vi "与其他模块交互 (子VI).vi"() -> ()   [LabVIEW 2016, in "质控单元.lvlib"]
uses:
  <vilib>/Plasmionique/MB Master/MB_Master_TCP/MB_Master_TCP.lvclass
  D:/Program Files (x86)/National Instruments/LabVIEW 2016/vi.lib/Plasmionique/MB Master/MB_Master/MB_Master.lvclass
  <vilib>/Plasmionique/MB Master/MB_Master/MB_Master.lvclass
  <vilib>/Plasmionique/MB Master/MB Master.lvlib
panel:
  in  "starting address 6":u16
  in  "values 6":u16[](array[numeric])
  in  "starting address 5":u16
  in  "values 5":u16[](array[numeric])
  in  "starting address 4":u16
  in  "values 4":u16[](array[numeric])
  in  "starting address 3":u16
  in  "values 3":u16[](array[numeric])
  in  "starting address 2":u16
  in  "values 2":u16[](array[numeric])
  in  "values":u16[](array[numeric])
  in  "starting address":u16
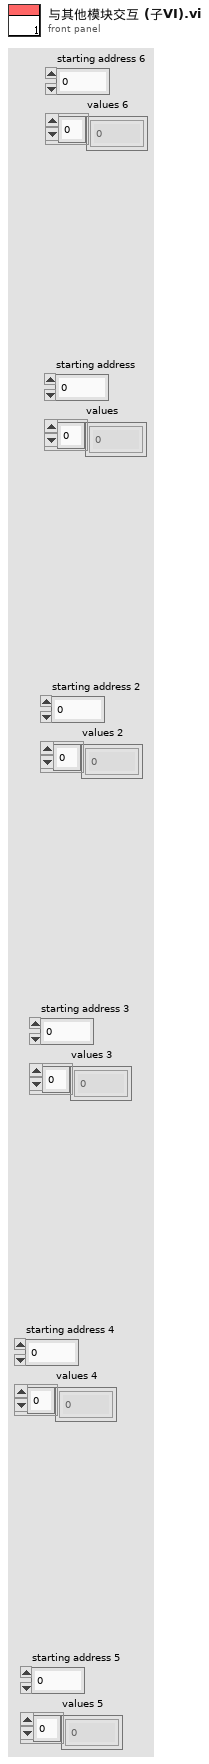
[diagram p1: front panel]
types:
  T1 = cluster{"因子编码":u32, "单位":u16, "标样参考值":sgl, "水样数据时间":timestamp, "水样实测值":sgl, "水样数据标识":string, "标样数据时间":timestamp, "标样实测值":sgl, "标样数据标识":string, "空白数据时间":timestamp, "空白实测值":sgl, "空白数据标识":string, "零点核查数据时间":timestamp, "零点核查实测值":sgl, "零点核查数据标识":string, "跨度核查数据时间":timestamp, "跨度核查实测值":sgl, "跨度核查数据标识":string, "加标回收数据时间":timestamp, "加标回收实测值":sgl, "加标回收数据标识":string, "平行样数据时间":timestamp, "平行样实测值":sgl, "平行样数据标识":string}
  T2 = cluster{"系统时间":timestamp, "工作状态":enum16{"空闲", "水样测试", "标样核查", "零点核查", "跨度核查", "空白测试", "平行样测试", "加标回收", "空白校准", "标样校准", "初始化（清洗）"}, "测量模式":enum16{"待机", "连续模式", "周期模式", "定点模式", "受控模式", "手动模式"}, "告警代码":enum16{"无告警", "缺试剂告警", "缺水样告警", "缺蒸馏水告警", "缺标液告警", "仪表漏液告警", "标定异常告警", "超量程告警", "加热异常", "低试剂预警", "超上限告警", "超下限告警", "仪表内部其他异常", "滴定异常告警", "电极异常告警", "量程切换告警", "参数设置告警", "PH电极电位异常", "电导率电极异常", "浊度光度异常", "溶解氧电极异常", "溶解氧光强异常", "温度异常告警", "PH异常告警", "溶解氧异常告警", "电导率异常告警", "浊度异常告警", "叶绿素异常告警", "藻密度异常告警", "蓝绿藻异常告警", "ORP异常告警", "氨氮异常告警", "清洁刷异常告警", "SD卡异常告警", "蓝牙异常告警", "Wifi异常告警", "流程异常告警"}, "故障代码":enum16{"无故障", "电机故障", "温度故障", "通讯故障", "滴定故障"}, "日志代码":u16, "软件版本":u16, "F0":sgl, "F1":sgl, "F2":sgl, "F3":sgl, "T":sgl, "H":sgl, "id":u16, "flowid":u16, "量程":u16, "总磷控温温度1":sgl, "营养盐控温温度2":sgl, "ADC":sgl}
  T3 = cluster{"Registers[0]":u16, "Registers[1]":u16, "Registers[2]":u16, "Registers[3]":u16, "Registers[4]":u16, "Registers[5]":u16, "Registers[6]":u16, "Registers[7]":u16, "Registers[8]":u16, "Registers[9]":u16, "Registers[10]":u16, "Registers[11]":u16, "Registers[12]":u16, "Registers[13]":u16, "Registers[14]":u16, "Registers[15]":u16, "Registers[16]":u16, "Registers[17]":u16, "Registers[18]":u16, "Registers[19]":u16, "Registers[20]":u16, "Registers[21]":u16, "Registers[22]":u16, "Registers[23]":u16, "Registers[24]":u16, "Registers[25]":u16, "Registers[26]":u16, "Registers[27]":u16, "Registers[28]":u16, "Registers[29]":u16, "Registers[30]":u16, "Registers[31]":u16, "Registers[32]":u16, "Registers[33]":u16, "Registers[34]":u16, "Registers[35]":u16, "Registers[36]":u16, "Registers[37]":u16, "Registers[38]":u16, "Registers[39]":u16, "Registers[40]":u16, "Registers[41]":u16, "Registers[42]":u16, "Registers[43]":u16, "Registers[44]":u16, "Registers[45]":u16, "Registers[46]":u16, "Registers[47]":u16, "Registers[48]":u16, "Registers[49]":u16, "Registers[50]":u16, "Registers[51]":u16, "Registers[52]":u16, "Registers[53]":u16, "Registers[54]":u16, "Registers[55]":u16, "Registers[56]":u16}
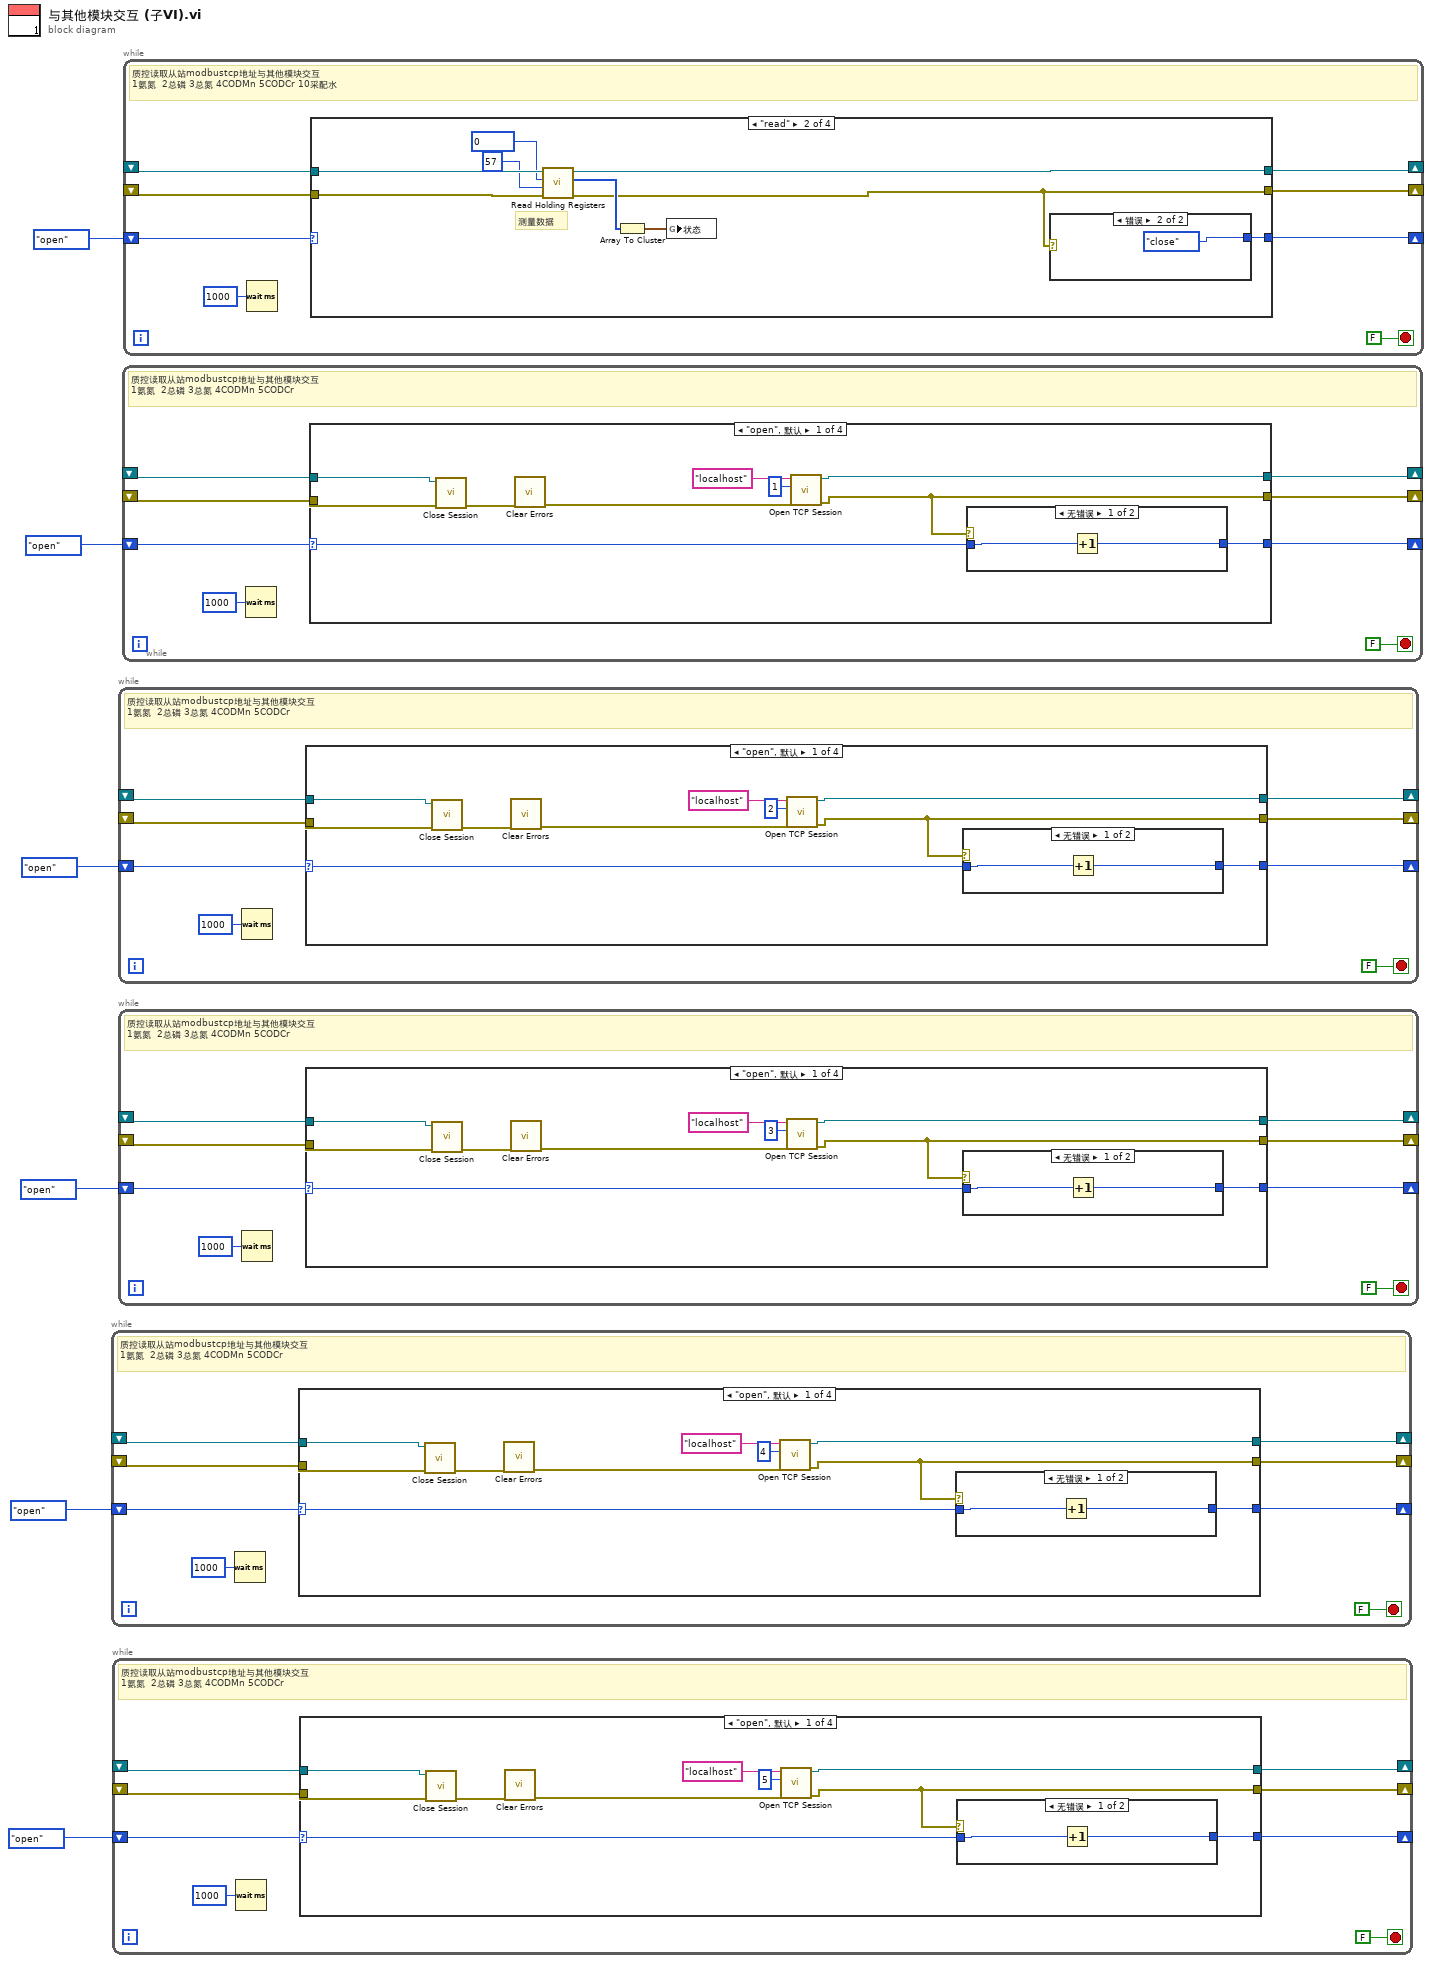
[diagram p0: block diagram]
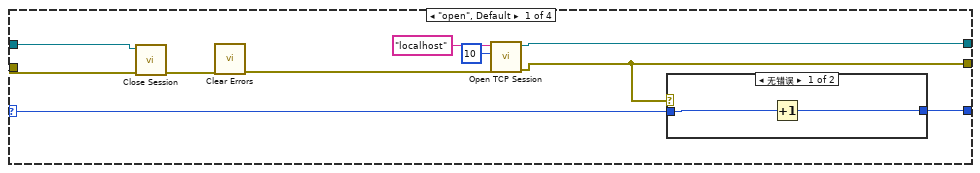
[diagram p2: hidden frame]
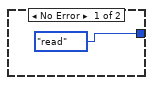
[diagram p4: hidden frame]
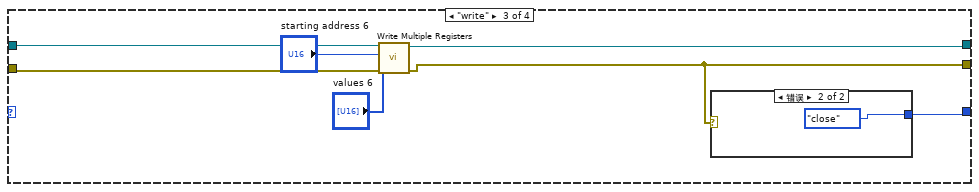
[diagram p5: hidden frame]
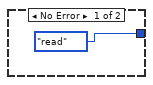
[diagram p6: hidden frame]
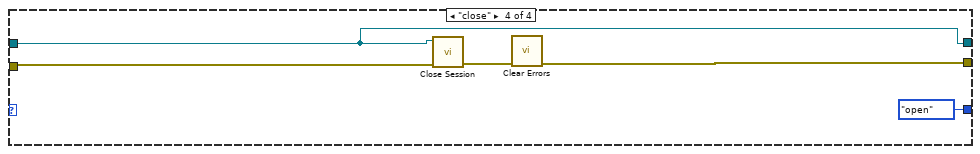
[diagram p7: hidden frame]
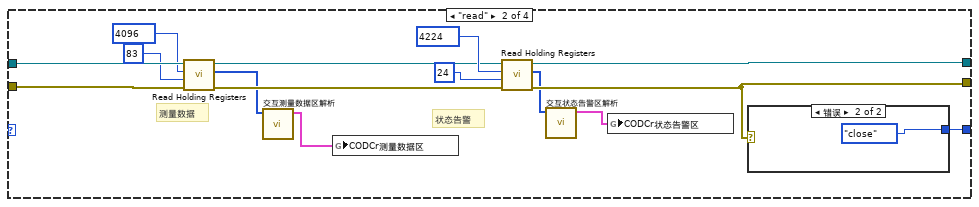
[diagram p9: hidden frame]
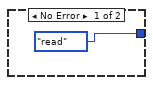
[diagram p10: hidden frame]
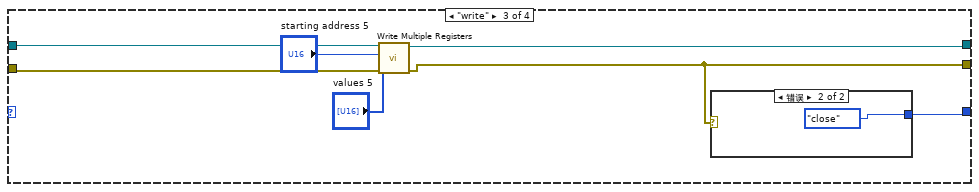
[diagram p11: hidden frame]
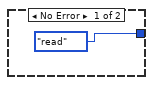
[diagram p12: hidden frame]
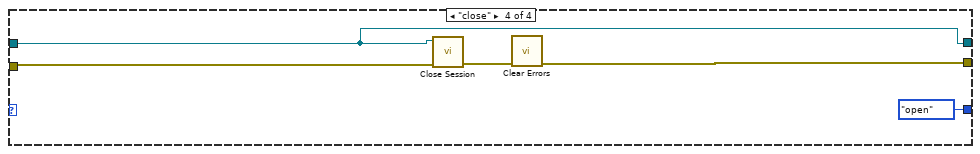
[diagram p13: hidden frame]
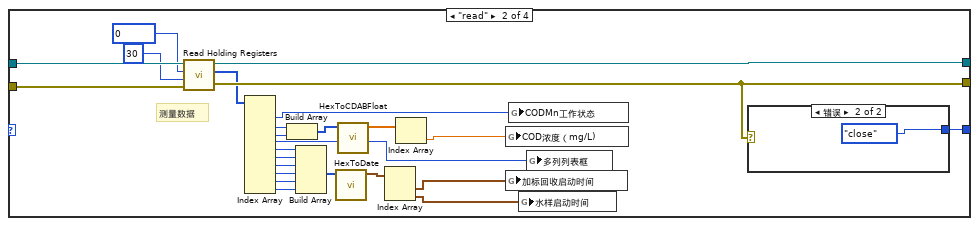
[diagram p15: hidden frame]
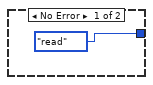
[diagram p16: hidden frame]
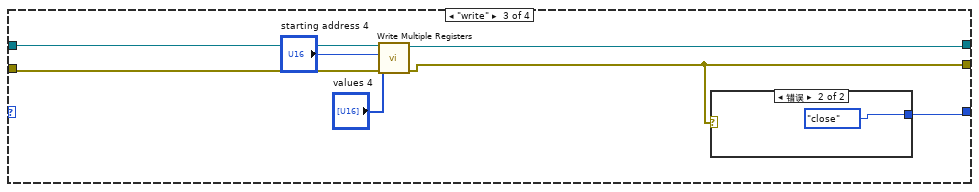
[diagram p17: hidden frame]
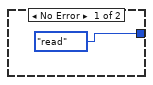
[diagram p18: hidden frame]
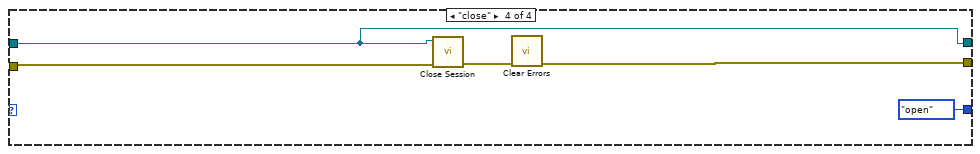
[diagram p19: hidden frame]
diagram:
  n1 = while {
    shift-right: [w12] -> _
    shift-left: _ -> [w14]
    shift-right: [w11] -> _
    shift-left: _ -> [w13]
    shift-right: [w8] -> _
    shift-left: enum16{"open", "read", "write", "close"}."open" -> [w9]
    stop <- FALSE stop-if-true
    # "质控读取从站modbustcp地址与其他模块交互\n1氨氮  2总磷 3总氮 4CODMn 5CODCr"
    n2 = Wait (ms)(milliseconds to wait=u32 1000 ("等待时间（毫秒）")) -> ()  [unwired: 1 out]
    n3 = case shown="\"open\", 默认" w9 {
      selector: w9 -> [w16 _ _ _]
      tunnel: w14 -> [w21 w52 w60 w68]
      tunnel: w13 -> [w20 w49 w59 w67]
      tunnel: [w22 w47 w58 w68] -> w12
      tunnel: [w17 w46 w57 w65] -> w11
      tunnel: [w15 w48 w61 enum16{"open", "read", "write", "close"}."open"] -> w8
      frame "open", Default {
        n4 = call-dynamic "Close Session.vi"("error in (no error)"=w20, "MB session in"=w21) -> ("error out"=w19:errorcluster)  [unwired: 9 in]
        n5 = call <vilib>:"Clear Errors.vi"("error in (no error)"=w19) -> ("error out"=w18:errorcluster)  [unwired: 5 in, 1 out]
        n6 = call <vilib>:"Open TCP Session.vi"("error in (no error)"=w18, "Port (502)"=u16 4, "IP Address"="localhost") -> ("error out"=w17:errorcluster, "MB_TCP session"=w22:refnum<class "MB_Master_TCP.lvclass">)  [unwired: 7 in]
        n7 = case shown="无错误" w17 {
          tunnel: w16 -> [w26 w27]
          tunnel: [w25 w27] -> w15
          frame No Error {
            n8 = Increment(x=w26) -> (x+1=w25:enum16{"open", "read", "write", "close"})
          }
          frame Error {
          }
        }
      }
      frame "read" {
        # "测量数据"
        n9 = call <vilib>:"Read Holding Registers.vi"("error in (no error)"=w49, "quantity"=u16 30, "starting address"=u16 0, "MB session in"=w52) -> ("error out"=w46:errorcluster, "Registers"=w45:u16[], "MB session out"=w47:refnum<class "MB_Master.lvclass">)  [unwired: 5 in]
        n10 = Index Array(array=w45) -> (element #1=w44:u16, element #2=w43:u16, element #3=w42:u16, element #4=w38:u16, element #5=w37:u16, element #6=w36:u16, element #7=w35:u16, element #8=w33:u16, element #9=w32:u16, element #10=w31:u16)  [unwired: 10 in]
        n11 = Build Array(w43, w42) -> (w41:u16[])
        n12 = Build Array(w37, w36, w35, w33, w32, w31) -> (w34:u16[])
        n13 = call "HexToDate.vi"("数组"=w34) -> ("DATE"=w30:timestamp[])  [unwired: 10 in]
        n14 = call "HexToCDABFloat.vi"("数组"=w41) -> ("FLOAT"=w40:sgl[])  [unwired: 10 in]
        n15 = Index Array(array=w30) -> (element #1=w29:timestamp, element #2=w28:timestamp)  [unwired: 2 in]
        n16 = Index Array(array=w40) -> (element=w39:sgl)  [unwired: 1 in]
        n17 = global write "与CODMn交互全局.vi" "COD浓度（mg/L)"(w39) -> ()
        n18 = global write "与CODMn交互全局.vi" "加标回收启动时间"(w29) -> ()
        n19 = global write "与CODMn交互全局.vi" "CODMn工作状态"(w44) -> ()
        n20 = global write "与CODMn交互全局.vi" "水样启动时间"(w28) -> ()
        n21 = global write "与CODMn交互全局.vi" "多列列表框"(w38) -> ()
        n22 = case shown="错误" w46 {
          tunnel: [enum16{"open", "read", "write", "close"}."read" enum16{"open", "read", "write", "close"}."close"] -> w48
          frame No Error {
          }
          frame Error {
          }
        }
      }
      frame "write" {
        n23 = call <vilib>:"Write Multiple Registers.vi"("error in (no error)"=w59, "values"="values 4", "starting address"="starting address 4", "MB session in"=w60) -> ("error out"=w57:errorcluster, "MB session out"=w58:refnum<class "MB_Master.lvclass">)  [unwired: 6 in]
        n24 = case shown="错误" w57 {
          tunnel: [enum16{"open", "read", "write", "close"}."read" enum16{"open", "read", "write", "close"}."close"] -> w61
          frame No Error {
          }
          frame Error {
          }
        }
      }
      frame "close" {
        n25 = call-dynamic "Close Session.vi"("error in (no error)"=w67, "MB session in"=w68) -> ("error out"=w66:errorcluster)  [unwired: 9 in]
        n26 = call <vilib>:"Clear Errors.vi"("error in (no error)"=w66) -> ("error out"=w65:errorcluster)  [unwired: 5 in, 1 out]
      }
    }
  }
  n27 = while {
    shift-right: [w74] -> _
    shift-left: _ -> [w76]
    shift-right: [w73] -> _
    shift-left: _ -> [w75]
    shift-right: [w70] -> _
    shift-left: enum16{"open", "read", "write", "close"}."open" -> [w71]
    stop <- FALSE stop-if-true
    # "质控读取从站modbustcp地址与其他模块交互\n1氨氮  2总磷 3总氮 4CODMn 5CODCr"
    n28 = Wait (ms)(milliseconds to wait=u32 1000 ("等待时间（毫秒）")) -> ()  [unwired: 1 out]
    n29 = case shown="\"open\", 默认" w71 {
      selector: w71 -> [w78 _ _ _]
      tunnel: w76 -> [w83 w104 w112 w120]
      tunnel: w75 -> [w82 w101 w111 w119]
      tunnel: [w84 w95 w110 w120] -> w74
      tunnel: [w79 w94 w109 w117] -> w73
      tunnel: [w77 w100 w113 enum16{"open", "read", "write", "close"}."open"] -> w70
      frame "open", Default {
        n30 = call-dynamic "Close Session.vi"("error in (no error)"=w82, "MB session in"=w83) -> ("error out"=w81:errorcluster)  [unwired: 9 in]
        n31 = call <vilib>:"Clear Errors.vi"("error in (no error)"=w81) -> ("error out"=w80:errorcluster)  [unwired: 5 in, 1 out]
        n32 = call <vilib>:"Open TCP Session.vi"("error in (no error)"=w80, "Port (502)"=u16 5, "IP Address"="localhost") -> ("error out"=w79:errorcluster, "MB_TCP session"=w84:refnum<class "MB_Master_TCP.lvclass">)  [unwired: 7 in]
        n33 = case shown="无错误" w79 {
          tunnel: w78 -> [w88 w89]
          tunnel: [w87 w89] -> w77
          frame No Error {
            n34 = Increment(x=w88) -> (x+1=w87:enum16{"open", "read", "write", "close"})
          }
          frame Error {
          }
        }
      }
      frame "read" {
        # "状态告警"
        # "测量数据"
        n35 = call <vilib>:"Read Holding Registers.vi"("error in (no error)"=w101, "quantity"=u16 83, "starting address"=u16 4096, "MB session in"=w104) -> ("error out"=w96:errorcluster, "Registers"=w93:u16[], "MB session out"=w97:refnum<class "MB_Master.lvclass">)  [unwired: 5 in]
        n36 = call "交互测量数据区解析.vi"("数组"=w93) -> ("测量数据区"=w91:T1)  [unwired: 10 in]
        n37 = global write "与CODCr交互全局.vi" "CODCr测量数据区"(w91) -> ()
        n38 = call <vilib>:"Read Holding Registers.vi"("error in (no error)"=w96, "quantity"=u16 24, "starting address"=u16 4224, "MB session in"=w97) -> ("error out"=w94:errorcluster, "Registers"=w92:u16[], "MB session out"=w95:refnum<class "MB_Master.lvclass">)  [unwired: 5 in]
        n39 = call "交互状态告警区解析.vi"("数组"=w92) -> ("状态告警区"=w90:T2)  [unwired: 10 in]
        n40 = global write "与CODCr交互全局.vi" "CODCr状态告警区"(w90) -> ()
        n41 = case shown="错误" w94 {
          tunnel: [enum16{"open", "read", "write", "close"}."read" enum16{"open", "read", "write", "close"}."close"] -> w100
          frame No Error {
          }
          frame Error {
          }
        }
      }
      frame "write" {
        n42 = call <vilib>:"Write Multiple Registers.vi"("error in (no error)"=w111, "values"="values 5", "starting address"="starting address 5", "MB session in"=w112) -> ("error out"=w109:errorcluster, "MB session out"=w110:refnum<class "MB_Master.lvclass">)  [unwired: 6 in]
        n43 = case shown="错误" w109 {
          tunnel: [enum16{"open", "read", "write", "close"}."read" enum16{"open", "read", "write", "close"}."close"] -> w113
          frame No Error {
          }
          frame Error {
          }
        }
      }
      frame "close" {
        n44 = call-dynamic "Close Session.vi"("error in (no error)"=w119, "MB session in"=w120) -> ("error out"=w118:errorcluster)  [unwired: 9 in]
        n45 = call <vilib>:"Clear Errors.vi"("error in (no error)"=w118) -> ("error out"=w117:errorcluster)  [unwired: 5 in, 1 out]
      }
    }
  }
  n46 = while {
    shift-right: [w126] -> _
    shift-left: _ -> [w128]
    shift-right: [w125] -> _
    shift-left: _ -> [w127]
    shift-right: [w122] -> _
    shift-left: enum16{"open", "read", "write", "close"}."open" -> [w123]
    stop <- FALSE stop-if-true
    # "质控读取从站modbustcp地址与其他模块交互\n1氨氮  2总磷 3总氮 4CODMn 5CODCr"
    n47 = Wait (ms)(milliseconds to wait=u32 1000 ("等待时间（毫秒）")) -> ()  [unwired: 1 out]
    n48 = case shown="\"open\", 默认" w123 {
      selector: w123 -> [w130 _ _ _]
      tunnel: w128 -> [w135 w156 w164 w172]
      tunnel: w127 -> [w134 w153 w163 w171]
      tunnel: [w136 w147 w162 w172] -> w126
      tunnel: [w131 w146 w161 w169] -> w125
      tunnel: [w129 w152 w165 enum16{"open", "read", "write", "close"}."open"] -> w122
      frame "open", Default {
        n49 = call-dynamic "Close Session.vi"("error in (no error)"=w134, "MB session in"=w135) -> ("error out"=w133:errorcluster)  [unwired: 9 in]
        n50 = call <vilib>:"Clear Errors.vi"("error in (no error)"=w133) -> ("error out"=w132:errorcluster)  [unwired: 5 in, 1 out]
        n51 = call <vilib>:"Open TCP Session.vi"("error in (no error)"=w132, "Port (502)"=u16 2, "IP Address"="localhost") -> ("error out"=w131:errorcluster, "MB_TCP session"=w136:refnum<class "MB_Master_TCP.lvclass">)  [unwired: 7 in]
        n52 = case shown="无错误" w131 {
          tunnel: w130 -> [w140 w141]
          tunnel: [w139 w141] -> w129
          frame No Error {
            n53 = Increment(x=w140) -> (x+1=w139:enum16{"open", "read", "write", "close"})
          }
          frame Error {
          }
        }
      }
      frame "read" {
        # "状态告警"
        # "测量数据"
        n54 = call <vilib>:"Read Holding Registers.vi"("error in (no error)"=w153, "quantity"=u16 83, "starting address"=u16 4096, "MB session in"=w156) -> ("error out"=w148:errorcluster, "Registers"=w145:u16[], "MB session out"=w149:refnum<class "MB_Master.lvclass">)  [unwired: 5 in]
        n55 = call "交互测量数据区解析.vi"("数组"=w145) -> ("测量数据区"=w143:T1)  [unwired: 10 in]
        n56 = global write "与总磷交互全局.vi" "总磷测量数据区"(w143) -> ()
        n57 = call <vilib>:"Read Holding Registers.vi"("error in (no error)"=w148, "quantity"=u16 24, "starting address"=u16 4224, "MB session in"=w149) -> ("error out"=w146:errorcluster, "Registers"=w144:u16[], "MB session out"=w147:refnum<class "MB_Master.lvclass">)  [unwired: 5 in]
        n58 = call "交互状态告警区解析.vi"("数组"=w144) -> ("状态告警区"=w142:T2)  [unwired: 10 in]
        n59 = global write "与总磷交互全局.vi" "总磷状态告警区"(w142) -> ()
        n60 = case shown="错误" w146 {
          tunnel: [enum16{"open", "read", "write", "close"}."read" enum16{"open", "read", "write", "close"}."close"] -> w152
          frame No Error {
          }
          frame Error {
          }
        }
      }
      frame "write" {
        n61 = call <vilib>:"Write Multiple Registers.vi"("error in (no error)"=w163, "values"="values 2", "starting address"="starting address 2", "MB session in"=w164) -> ("error out"=w161:errorcluster, "MB session out"=w162:refnum<class "MB_Master.lvclass">)  [unwired: 6 in]
        n62 = case shown="错误" w161 {
          tunnel: [enum16{"open", "read", "write", "close"}."read" enum16{"open", "read", "write", "close"}."close"] -> w165
          frame No Error {
          }
          frame Error {
          }
        }
      }
      frame "close" {
        n63 = call-dynamic "Close Session.vi"("error in (no error)"=w171, "MB session in"=w172) -> ("error out"=w170:errorcluster)  [unwired: 9 in]
        n64 = call <vilib>:"Clear Errors.vi"("error in (no error)"=w170) -> ("error out"=w169:errorcluster)  [unwired: 5 in, 1 out]
      }
    }
  }
  n65 = while {
    shift-right: [w178] -> _
    shift-left: _ -> [w180]
    shift-right: [w177] -> _
    shift-left: _ -> [w179]
    shift-right: [w174] -> _
    shift-left: enum16{"open", "read", "write", "close"}."open" -> [w175]
    stop <- FALSE stop-if-true
    # "质控读取从站modbustcp地址与其他模块交互\n1氨氮  2总磷 3总氮 4CODMn 5CODCr"
    n66 = Wait (ms)(milliseconds to wait=u32 1000 ("等待时间（毫秒）")) -> ()  [unwired: 1 out]
    n67 = case shown="\"open\", 默认" w175 {
      selector: w175 -> [w182 _ _ _]
      tunnel: w180 -> [w187 w208 w216 w224]
      tunnel: w179 -> [w186 w205 w215 w223]
      tunnel: [w188 w199 w214 w224] -> w178
      tunnel: [w183 w198 w213 w221] -> w177
      tunnel: [w181 w204 w217 enum16{"open", "read", "write", "close"}."open"] -> w174
      frame "open", Default {
        n68 = call-dynamic "Close Session.vi"("error in (no error)"=w186, "MB session in"=w187) -> ("error out"=w185:errorcluster)  [unwired: 9 in]
        n69 = call <vilib>:"Clear Errors.vi"("error in (no error)"=w185) -> ("error out"=w184:errorcluster)  [unwired: 5 in, 1 out]
        n70 = call <vilib>:"Open TCP Session.vi"("error in (no error)"=w184, "Port (502)"=u16 3, "IP Address"="localhost") -> ("error out"=w183:errorcluster, "MB_TCP session"=w188:refnum<class "MB_Master_TCP.lvclass">)  [unwired: 7 in]
        n71 = case shown="无错误" w183 {
          tunnel: w182 -> [w192 w193]
          tunnel: [w191 w193] -> w181
          frame No Error {
            n72 = Increment(x=w192) -> (x+1=w191:enum16{"open", "read", "write", "close"})
          }
          frame Error {
          }
        }
      }
      frame "read" {
        # "状态告警"
        # "测量数据"
        n73 = call <vilib>:"Read Holding Registers.vi"("error in (no error)"=w205, "quantity"=u16 83, "starting address"=u16 4096, "MB session in"=w208) -> ("error out"=w200:errorcluster, "Registers"=w197:u16[], "MB session out"=w201:refnum<class "MB_Master.lvclass">)  [unwired: 5 in]
        n74 = call "交互测量数据区解析.vi"("数组"=w197) -> ("测量数据区"=w195:T1)  [unwired: 10 in]
        n75 = global write "与总氮交互全局.vi" "总氮测量数据区"(w195) -> ()
        n76 = call <vilib>:"Read Holding Registers.vi"("error in (no error)"=w200, "quantity"=u16 24, "starting address"=u16 4224, "MB session in"=w201) -> ("error out"=w198:errorcluster, "Registers"=w196:u16[], "MB session out"=w199:refnum<class "MB_Master.lvclass">)  [unwired: 5 in]
        n77 = call "交互状态告警区解析.vi"("数组"=w196) -> ("状态告警区"=w194:T2)  [unwired: 10 in]
        n78 = global write "与总氮交互全局.vi" "总氮状态告警区"(w194) -> ()
        n79 = case shown="错误" w198 {
          tunnel: [enum16{"open", "read", "write", "close"}."read" enum16{"open", "read", "write", "close"}."close"] -> w204
          frame No Error {
          }
          frame Error {
          }
        }
      }
      frame "write" {
        n80 = call <vilib>:"Write Multiple Registers.vi"("error in (no error)"=w215, "values"="values 3", "starting address"="starting address 3", "MB session in"=w216) -> ("error out"=w213:errorcluster, "MB session out"=w214:refnum<class "MB_Master.lvclass">)  [unwired: 6 in]
        n81 = case shown="错误" w213 {
          tunnel: [enum16{"open", "read", "write", "close"}."read" enum16{"open", "read", "write", "close"}."close"] -> w217
          frame No Error {
          }
          frame Error {
          }
        }
      }
      frame "close" {
        n82 = call-dynamic "Close Session.vi"("error in (no error)"=w223, "MB session in"=w224) -> ("error out"=w222:errorcluster)  [unwired: 9 in]
        n83 = call <vilib>:"Clear Errors.vi"("error in (no error)"=w222) -> ("error out"=w221:errorcluster)  [unwired: 5 in, 1 out]
      }
    }
  }
  n84 = while {
    shift-right: [w230] -> _
    shift-left: _ -> [w232]
    shift-right: [w229] -> _
    shift-left: _ -> [w231]
    shift-right: [w226] -> _
    shift-left: enum16{"open", "read", "write", "close"}."open" -> [w227]
    stop <- FALSE stop-if-true
    # "质控读取从站modbustcp地址与其他模块交互\n1氨氮  2总磷 3总氮 4CODMn 5CODCr"
    n85 = Wait (ms)(milliseconds to wait=u32 1000 ("等待时间（毫秒）")) -> ()  [unwired: 1 out]
    n86 = case shown="\"open\", 默认" w227 {
      selector: w227 -> [w234 _ _ _]
      tunnel: w232 -> [w239 w260 w268 w276]
      tunnel: w231 -> [w238 w257 w267 w275]
      tunnel: [w240 w251 w266 w276] -> w230
      tunnel: [w235 w250 w265 w273] -> w229
      tunnel: [w233 w256 w269 enum16{"open", "read", "write", "close"}."open"] -> w226
      frame "open", Default {
        n87 = call-dynamic "Close Session.vi"("error in (no error)"=w238, "MB session in"=w239) -> ("error out"=w237:errorcluster)  [unwired: 9 in]
        n88 = call <vilib>:"Clear Errors.vi"("error in (no error)"=w237) -> ("error out"=w236:errorcluster)  [unwired: 5 in, 1 out]
        n89 = call <vilib>:"Open TCP Session.vi"("error in (no error)"=w236, "Port (502)"=u16 1, "IP Address"="localhost") -> ("error out"=w235:errorcluster, "MB_TCP session"=w240:refnum<class "MB_Master_TCP.lvclass">)  [unwired: 7 in]
        n90 = case shown="无错误" w235 {
          tunnel: w234 -> [w244 w245]
          tunnel: [w243 w245] -> w233
          frame No Error {
            n91 = Increment(x=w244) -> (x+1=w243:enum16{"open", "read", "write", "close"})
          }
          frame Error {
          }
        }
      }
      frame "read" {
        # "状态告警"
        # "测量数据"
        n92 = call <vilib>:"Read Holding Registers.vi"("error in (no error)"=w257, "quantity"=u16 83, "starting address"=u16 4096, "MB session in"=w260) -> ("error out"=w252:errorcluster, "Registers"=w249:u16[], "MB session out"=w253:refnum<class "MB_Master.lvclass">)  [unwired: 5 in]
        n93 = call "交互测量数据区解析.vi"("数组"=w249) -> ("测量数据区"=w248:T1)  [unwired: 10 in]
        n94 = global write "与氨氮交互全局.vi" "氨氮测量数据区"(w248) -> ()
        n95 = call <vilib>:"Read Holding Registers.vi"("error in (no error)"=w252, "quantity"=u16 24, "starting address"=u16 4224, "MB session in"=w253) -> ("error out"=w250:errorcluster, "Registers"=w247:u16[], "MB session out"=w251:refnum<class "MB_Master.lvclass">)  [unwired: 5 in]
        n96 = call "交互状态告警区解析.vi"("数组"=w247) -> ("状态告警区"=w246:T2)  [unwired: 10 in]
        n97 = global write "与氨氮交互全局.vi" "氨氮状态告警区"(w246) -> ()
        n98 = case shown="错误" w250 {
          tunnel: [enum16{"open", "read", "write", "close"}."read" enum16{"open", "read", "write", "close"}."close"] -> w256
          frame No Error {
          }
          frame Error {
          }
        }
      }
      frame "write" {
        n99 = call <vilib>:"Write Multiple Registers.vi"("error in (no error)"=w267, "values"="values", "starting address"="starting address", "MB session in"=w268) -> ("error out"=w265:errorcluster, "MB session out"=w266:refnum<class "MB_Master.lvclass">)  [unwired: 6 in]
        n100 = case shown="错误" w265 {
          tunnel: [enum16{"open", "read", "write", "close"}."read" enum16{"open", "read", "write", "close"}."close"] -> w269
          frame No Error {
          }
          frame Error {
          }
        }
      }
      frame "close" {
        n101 = call-dynamic "Close Session.vi"("error in (no error)"=w275, "MB session in"=w276) -> ("error out"=w274:errorcluster)  [unwired: 9 in]
        n102 = call <vilib>:"Clear Errors.vi"("error in (no error)"=w274) -> ("error out"=w273:errorcluster)  [unwired: 5 in, 1 out]
      }
    }
  }
  n103 = while {
    shift-right: [w282] -> _
    shift-left: _ -> [w284]
    shift-right: [w281] -> _
    shift-left: _ -> [w283]
    shift-right: [w278] -> _
    shift-left: enum16{"open", "read", "write", "close"}."open" -> [w279]
    stop <- FALSE stop-if-true
    # "质控读取从站modbustcp地址与其他模块交互\n1氨氮  2总磷 3总氮 4CODMn 5CODCr 10采配水"
    n104 = Wait (ms)(milliseconds to wait=u32 1000 ("等待时间（毫秒）")) -> ()  [unwired: 1 out]
    n105 = case shown="\"read\"" w279 {
      selector: w279 -> [w286 _ _ _]
      tunnel: w284 -> [w291 w306 w314 w322]
      tunnel: w283 -> [w290 w303 w313 w321]
      tunnel: [w292 w299 w312 w322] -> w282
      tunnel: [w287 w298 w311 w319] -> w281
      tunnel: [w285 w302 w315 enum16{"open", "read", "write", "close"}."open"] -> w278
      frame "open", Default {
        n106 = call-dynamic "Close Session.vi"("error in (no error)"=w290, "MB session in"=w291) -> ("error out"=w289:errorcluster)  [unwired: 9 in]
        n107 = call <vilib>:"Clear Errors.vi"("error in (no error)"=w289) -> ("error out"=w288:errorcluster)  [unwired: 5 in, 1 out]
        n108 = call <vilib>:"Open TCP Session.vi"("error in (no error)"=w288, "Port (502)"=u16 10, "IP Address"="localhost") -> ("error out"=w287:errorcluster, "MB_TCP session"=w292:refnum<class "MB_Master_TCP.lvclass">)  [unwired: 7 in]
        n109 = case shown="无错误" w287 {
          tunnel: w286 -> [w296 w297]
          tunnel: [w295 w297] -> w285
          frame No Error {
            n110 = Increment(x=w296) -> (x+1=w295:enum16{"open", "read", "write", "close"})
          }
          frame Error {
          }
        }
      }
      frame "read" {
        # "测量数据"
        n111 = call <vilib>:"Read Holding Registers.vi"("error in (no error)"=w303, "quantity"=u16 57, "starting address"=u16 0, "MB session in"=w306) -> ("error out"=w298:errorcluster, "Registers"=w301:u16[], "MB session out"=w299:refnum<class "MB_Master.lvclass">)  [unwired: 5 in]
        n112 = Array To Cluster(array=w301) -> (cluster=w300:T3)
        n113 = global write "与采配水交互全局.vi" "状态"(w300) -> ()
        n114 = case shown="错误" w298 {
          tunnel: [enum16{"open", "read", "write", "close"}."read" enum16{"open", "read", "write", "close"}."close"] -> w302
          frame No Error {
          }
          frame Error {
          }
        }
      }
      frame "write" {
        n115 = call <vilib>:"Write Multiple Registers.vi"("error in (no error)"=w313, "values"="values 6", "starting address"="starting address 6", "MB session in"=w314) -> ("error out"=w311:errorcluster, "MB session out"=w312:refnum<class "MB_Master.lvclass">)  [unwired: 6 in]
        n116 = case shown="错误" w311 {
          tunnel: [enum16{"open", "read", "write", "close"}."read" enum16{"open", "read", "write", "close"}."close"] -> w315
          frame No Error {
          }
          frame Error {
          }
        }
      }
      frame "close" {
        n117 = call-dynamic "Close Session.vi"("error in (no error)"=w321, "MB session in"=w322) -> ("error out"=w320:errorcluster)  [unwired: 9 in]
        n118 = call <vilib>:"Clear Errors.vi"("error in (no error)"=w320) -> ("error out"=w319:errorcluster)  [unwired: 5 in, 1 out]
      }
    }
  }
